vi "createCommandList.vi"(8 "error in (no error)":errorcluster, 10 "Parameters":u32[](array[numeric]), 11 "Surge in":refnum<class "Surge.lvclass">) -> (0 "error out":errorcluster, 2 "Commandlist":string, 3 "Surge out":refnum<class "Surge.lvclass">)   [LabVIEW 2013, in "Surge.lvclass"]
uses:
  Surge.lvclass
  lib/Utilities.lvlib
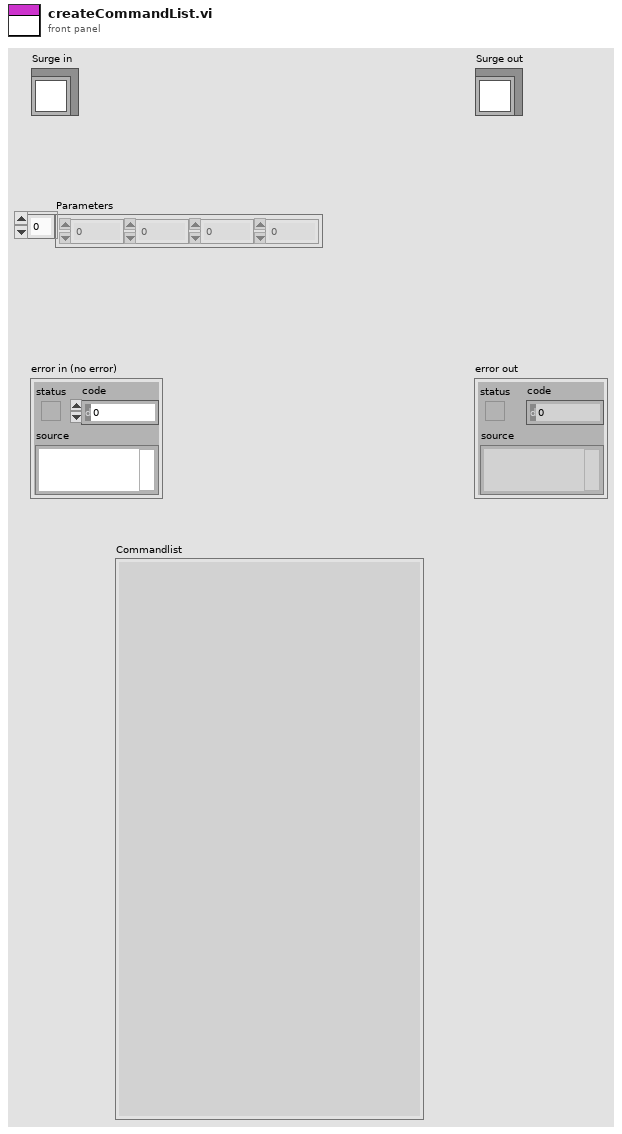
[diagram p1: front panel]
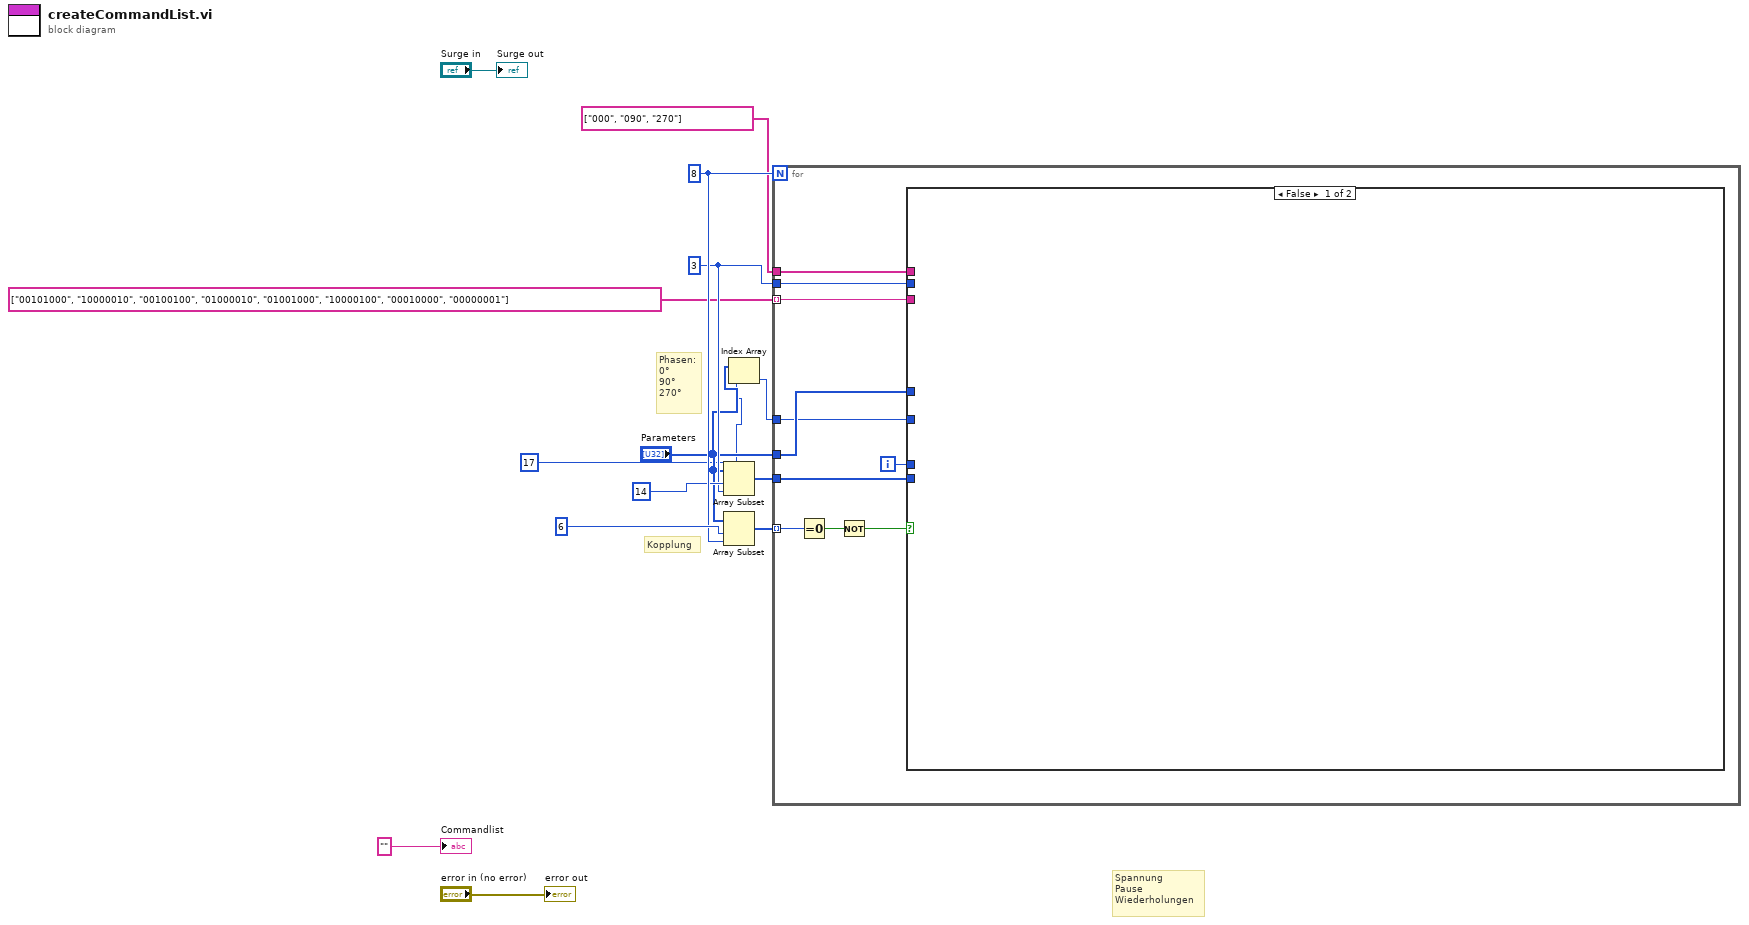
[diagram p0: block diagram]
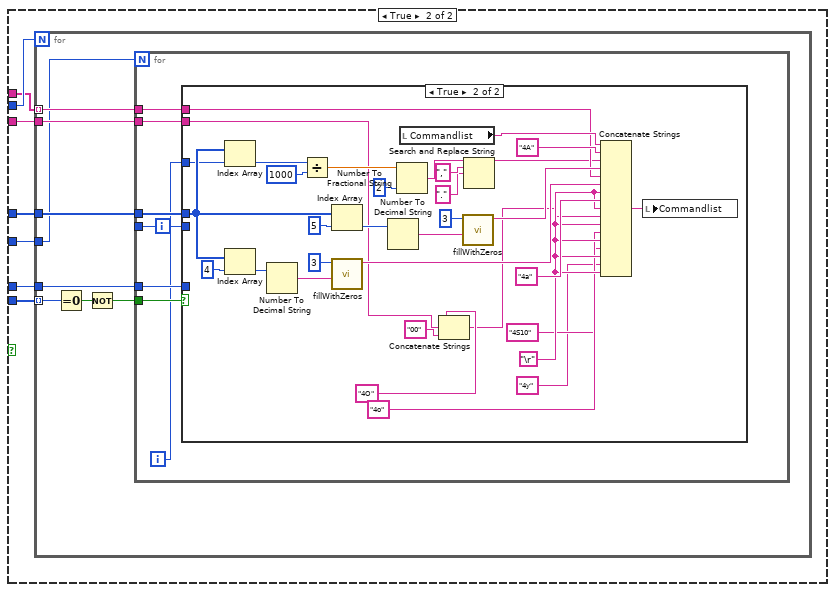
[diagram p2: hidden frame]
diagram:
  w9 = 3 ("length")
  w13 = 8 ("length")
  # "Kopplung"
  # "Spannung\nPause\nWiederholungen"
  # "Phasen:\n0°\n90°\n270°"
  n1 = Array Subset(array="Parameters", index=14, length=w9) -> (w10:u32[])
  n2 = Array Subset(array="Parameters", index=6, length=w13) -> (w12:u32[])
  n3 = Index Array(array="Parameters", index=17) -> (element=w1:u32)
  n4 = for {
    N: w13 -> [_]
    tunnel: w12 -> [w24] mode=indexing
    tunnel: w10 -> [w21]
    tunnel: w9 -> [w20]
    tunnel: "Parameters" -> [w19]
    tunnel: string[] ["000", "090", "270"] -> [w17]
    tunnel: string[] ["00101000", "10000010", "00100100", "01000010", "01001000", "10000100", "00010000", "00000001"] -> [w16] mode=indexing
    tunnel: w1 -> [w15]
    i -> [w18]
    n5 = Equal To 0?(x=w24) -> (x = 0?=w23:bool)
    n6 = Not(x=w23) -> (.not. x?=w22:bool)
    n7 = case shown="False" w22 {
      tunnel: w21 -> [_ w30]
      tunnel: w20 -> [_ w31]
      tunnel: w19 -> [_ w29]
      tunnel: w18 -> [_ w28]
      tunnel: w17 -> [_ w27]
      tunnel: w16 -> [_ w26]
      tunnel: w15 -> [_ w25]
      frame False {
      }
      frame True {
        n8 = for {
          N: w31 -> [_]
          tunnel: w30 -> [w37] mode=indexing
          tunnel: w29 -> [w38]
          tunnel: w28 -> [w35]
          tunnel: w27 -> [w34] mode=indexing
          tunnel: w26 -> [w33]
          tunnel: w25 -> [w32]
          i -> [w36]
          n9 = Equal To 0?(x=w37) -> (x = 0?=w40:bool)
          n10 = Not(x=w40) -> (.not. x?=w39:bool)
          n11 = for {
            N: w32 -> [_]
            tunnel: w39 -> [w47]
            tunnel: w38 -> [w46]
            tunnel: w36 -> [w45]
            tunnel: w35 -> [w44]
            tunnel: w34 -> [w43]
            tunnel: w33 -> [w42]
            i -> [w41]
            n12 = case shown="True" w47 {
              tunnel: w46 -> [_ w76]
              tunnel: w45 -> [_ _]
              tunnel: w44 -> [_ _]
              tunnel: w43 -> [_ w63]
              tunnel: w42 -> [_ w55]
              tunnel: w41 -> [_ w48]
              frame False {
              }
              frame True {
                w56 = "\r"
                n13 = Index Array(array=w76, index=w48) -> (element=w75:u32)
                n14 = Index Array(array=w76, index=4) -> (element=w66:u32)
                n15 = Number To Decimal String(number=w66) -> (decimal integer string=w64:string)  [unwired: 1 in]
                n16 = Divide(x=w75, y=u32 1000) -> (x/y=w73:dbl)
                n17 = Index Array(array=w76, index=5) -> (element=w69:u32)
                n18 = call "fillWithZeros.vi"("string in"=w64, "width"=3) -> ("string out"=w62:string)  [unwired: 9 in]
                n19 = Number To Decimal String(number=w69) -> (decimal integer string=w68:string)  [unwired: 1 in]
                n20 = Number To Fractional String(number=w73, precision (6)=i16 2) -> (F-format string=w60:string)  [unwired: 2 in]
                n21 = local read "Commandlist"() -> (w79:string)
                n22 = Concatenate Strings("4O" ("string"), w55, "00" ("string")) -> (w52:string)
                n23 = call "fillWithZeros.vi"("string in"=w68, "width"=3) -> ("string out"=w67:string)  [unwired: 9 in]
                n24 = Search and Replace String(input string=w60, search string=",", replace string="." ("replace string (\"\")")) -> (result string=w57:string)  [unwired: 5 in, 3 out]
                n25 = Concatenate Strings(w79, "4A" ("string"), w57, w67, w63, w62, w56, "4a" ("string"), w56, w52, w56, "4o" ("string"), w56, "4S10" ("string"), w56, "4y" ("string"), w56) -> (w80:string)
                n26 = local write "Commandlist"(w80) -> ()
              }
            }
          }
        }
      }
    }
  }
  "error out" <- "error in (no error)"
  "Surge out" <- "Surge in"
  "Commandlist" <- ""
